vi "checksum.vi"(3 "Data":string) -> (0 "Check Sum":string, 1 "Data":string)   [LabVIEW 2009]
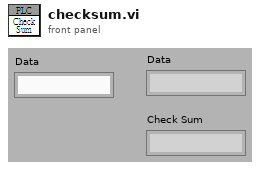
[diagram p1: front panel]
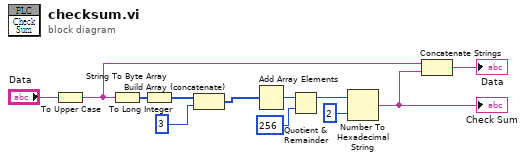
[diagram p0: block diagram]
diagram:
  n1 = To Upper Case(1:"Data") -> (0:w9:string)
  n2 = String To Byte Array(string=w9) -> (unsigned byte array=w4:u8[])
  n3 = To Long Integer(number=w4) -> (32bit integer=w3:i32[])
  n4 = Build Array (concatenate)(w3, 3) -> (w2:i32[])
  n5 = Add Array Elements(numeric array=w2) -> (sum=w5:i32)
  n6 = Quotient & Remainder(x=w5, y=256) -> (x-y*floor(x/y)=w6:i32)  [unwired: 1 out]
  n7 = Number To Hexadecimal String(1:i16 2 ("width (-)"), 2:w6) -> (0:w7:string)
  "Check Sum" <- w7
  n8 = Concatenate Strings(w9, w7) -> (→"Data":string)
